vi "Haskel Fast Forward.vi"(4 "Time Target (s)":dbl=10.0 format="%#_13g", 5 "Init":bool, 7 "Direction":T1=enum."Chamber", 8 "error in (no error)":errorcluster, 11 "Stand in":refnum<class "Stand.lvclass">) -> (0 "error out":errorcluster, 2 "Done":bool caption="Time has Elapsed")   [LabVIEW 2019, in "Stand.lvclass"]
uses:
  Stand.lvclass
  D:/GIT H4000/H4000/src/Device_class/Device.lvclass
  TypeDef/Direction.ctl
  Device_class/Device.lvclass/Device.ctl
  Stand.lvclass/Stand.ctl
  AI_class/AI.lvclass/AI.ctl
  AnalogComparator_class/AnalogComparator.lvclass/AnalogComparator.ctl
  AnalogComparator_class/GetStatus.vi
  Global/Global Constant.vi
  <vilib>/addons/_JKI.lib/FPGA_Basic_Components/Counter_32bit JKI_FPGA.vi
  FPGA_API_class/FPGA API.lvclass
  Device_class/Device.lvclass
  AI_class/AI.lvclass
  <vilib>/addons/_JKI.lib/FPGA_Basic_Components/JKI_BasicFPGA_Functions JKI_FPGA.lvlib
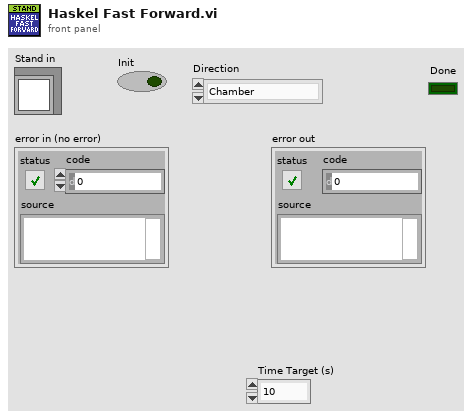
[diagram p1: front panel]
types:
  T1 = typedef "Direction.ctl" = enum8{"DUT", "Chamber"}
  T2 = typedef "AI_Data.ctl" = cluster{"Stat Data":T3, "OutOfRangeMax":bool, "OutOfRangeMin":bool, "HIHI":bool, "HI":bool, "LO":bool, "LOLO":bool}
  T3 = typedef "AI Statistics Data.ctl" = cluster{"raw mean":dbl, "scl mean":dbl, "raw mean 1Hz":dbl, "scl mean 1Hz":dbl}
  T4 = typedef "Setting Pressure PI.ctl" = cluster{"A [MPa/V]":dbl, "P0 [MPa]":dbl}
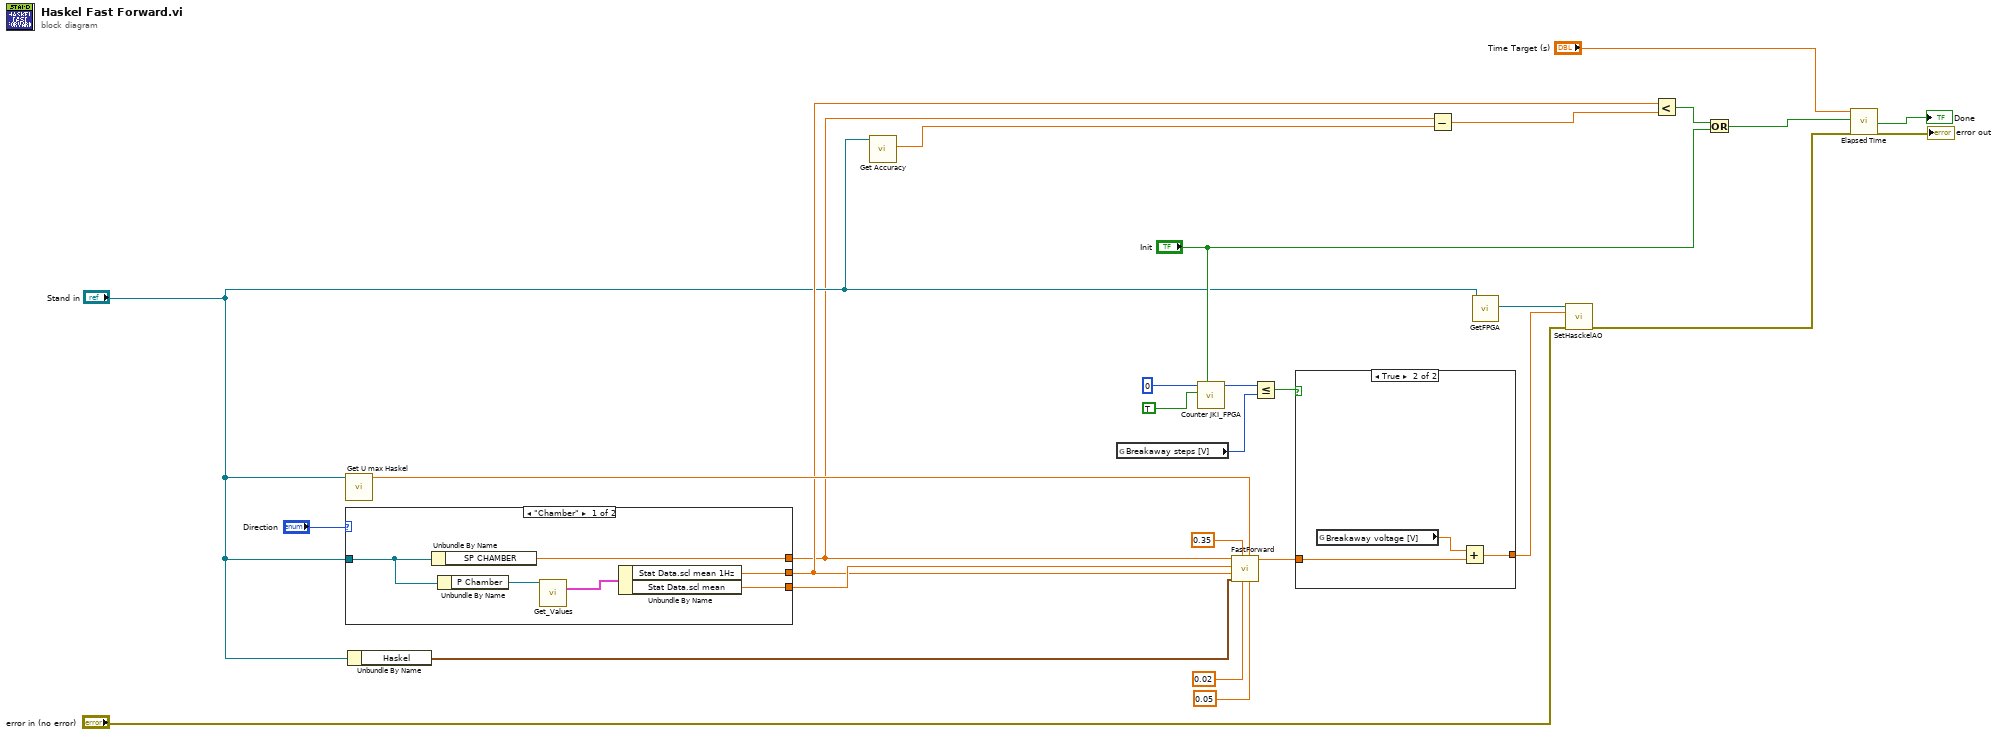
[diagram p0: block diagram]
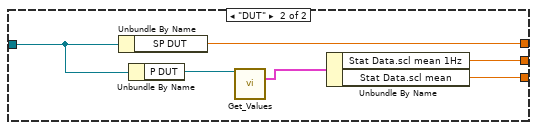
[diagram p3: hidden frame]
diagram:
  n1 = call "Get U max Haskel.vi"("Stand in"="Stand in") -> ("U max [V]"=w9:dbl)  [unwired: 10 in]
  n2 = case shown="\"Chamber\"" "Direction" {
    tunnel: [w34 w40] -> w21
    tunnel: [w29 w38] -> w1
    tunnel: "Stand in" -> [w32 w37]
    tunnel: [w30 w35] -> w4
    frame "Chamber" {
      n3 = Unbundle By Name(w32) -> ("SP CHAMBER"=w29:dbl)
      n4 = Unbundle By Name(w32) -> ("P Chamber"=w31:refnum<class "AI.lvclass">)
      n5 = call "Get_Values.vi"("reference in"=w31) -> ("Data"=w33:T2)  [unwired: 14 in]
      n6 = Unbundle By Name(w33) -> ("Stat Data.scl mean 1Hz"=w30:dbl, "Stat Data.scl mean"=w34:dbl)
    }
    frame "DUT" {
      n7 = Unbundle By Name(w37) -> ("SP DUT"=w38:dbl)
      n8 = Unbundle By Name(w37) -> ("P DUT"=w36:refnum<class "AI.lvclass">)
      n9 = call "Get_Values.vi"("reference in"=w36) -> ("Data"=w39:T2)  [unwired: 14 in]
      n10 = Unbundle By Name(w39) -> ("Stat Data.scl mean 1Hz"=w35:dbl, "Stat Data.scl mean"=w40:dbl)
    }
  }
  n11 = Unbundle By Name("Stand in") -> ("Haskel"=w25:T4)
  n12 = call "Get Accuracy.vi"("Stand in"="Stand in") -> ("Accuracy [MPa]"=w2:dbl)  [unwired: 10 in]
  n13 = global read "Global Constant.vi" "Breakaway steps [V]"() -> (w10:u32)
  n14 = call-poly <vilib>:"Counter JKI_FPGA.vi"("Reset? (F)"="Init", "Count Up? (T)"=TRUE, "Initial Value in"=u32 0) -> ("Counter Out"=w11:u32)  [unwired: 8 in]
  n15 = call "FastForward.vi"("delta U [V]"=0.05, "U max [V]"=w9, "Epsilon A"=0.02, "U min [V]"=0.35, "Setting"=w25, "Mean"=w4, "PV"=w21, "SP"=w1) -> ("U"=w7:dbl)  [unwired: 3 in]
  n16 = Less Or Equal?(x=w11, y=w10) -> (x <= y?=w8:bool)
  n17 = case shown="True" w8 {
    tunnel: w7 -> [w41 w44]
    tunnel: [w41 w43] -> w6
    frame False {
    }
    frame True {
      n18 = global read "Global Constant.vi" "Breakaway voltage [V]"() -> (w42:dbl)
      n19 = Add(x=w42, y=w44) -> (x+y=w43:dbl)
    }
  }
  n20 = Subtract(x=w1, y=w2) -> (x-y=w5:dbl)
  n21 = call "GetFPGA.vi"("Device in"="Stand in") -> ("FPGA API.lvclass"=w24:refnum<class "FPGA API.lvclass">)  [unwired: 10 in]
  n22 = call-dynamic "SetHasckelAO.vi"("FPGA API in"=w24, "Haskel in"=w6, "error in (no error)"="error in (no error)") -> ("error out"=w17:errorcluster)  [unwired: 11 in, 1 out]
  n23 = Less?(x=w4, y=w5) -> (x < y?=w20:bool)
  n24 = Or(x=w20, y="Init") -> (x .or. y?=w15:bool)
  n25 = call "Elapsed Time"("Time Target (s)"="Time Target (s)", "Reset"=w15, "error in (no error)"=w17) -> ("Time has Elapsed"=→"Done":bool, "error out"=→"error out":errorcluster)  [unwired: 9 in, 6 out]
